vi "Get Symbol Handle.vi"(8 "error in (no error)":errorcluster, 10 "Symbol Name":string, 11 "TwinCAT ADS in":refnum<class "TwinCAT ADS.lvclass">) -> (0 "error out":errorcluster, 2 "Handle":i32=-1, 3 "TwinCAT ADS out":refnum<class "TwinCAT ADS.lvclass">)   [LabVIEW 2018, in "TwinCAT ADS.lvclass"]
uses:
  TwinCAT ADS.lvclass
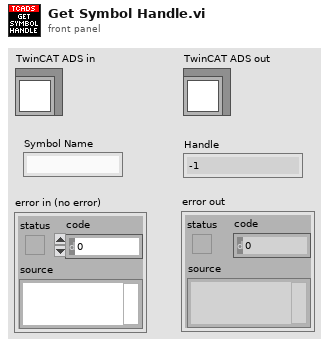
[diagram p1: front panel]
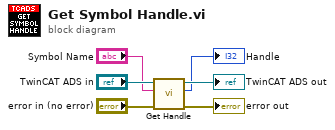
[diagram p0: block diagram]
diagram:
  n1 = call "Get Handle.vi"("error in (no error)"="error in (no error)", "Symbol Name"="Symbol Name", "TwinCAT ADS in"="TwinCAT ADS in") -> ("error out"=→"error out":errorcluster, "Handle"=→"Handle":i32, "TwinCAT ADS out"=→"TwinCAT ADS out":refnum<class "TwinCAT ADS.lvclass">)  [unwired: 6 in]
